vi "Build Error Message.vi"(8 "error IO":errorcluster, 9 "Enum":T1, 10 "Address":u8) -> (3 "Error Cluster":T2)   [LabVIEW 2015, in "J1939 Addon Shared.lvlib"]
uses:
  J1939 Addon Shared.lvlib
  Types/Error Cluster.ctl
  Types/Error Types.ctl
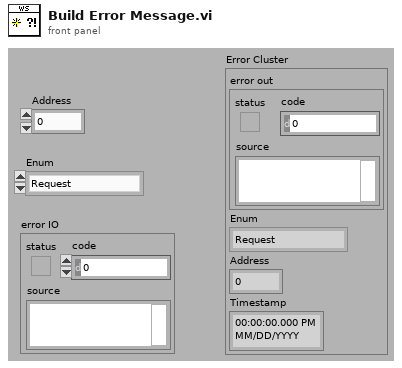
[diagram p1: front panel]
types:
  T1 = typedef "J1939 Addon Shared.lvlib/Error Types.ctl" = enum16{"Request", "RAW Generation", "Clear Active DTCs", "Clear Previous DTCs", "Addresses", "TLAs", "Get Active DTCs", "Get Previous DTCs", "TCP Connection"}
  T2 = typedef "J1939 Addon Shared.lvlib/Error Cluster.ctl" = cluster{"error out":errorcluster, "Enum":T1, "Address":u8, "Timestamp":timestamp}
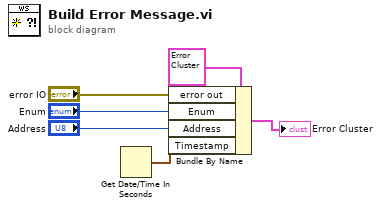
[diagram p0: block diagram]
diagram:
  n1 = Get Date/Time In Seconds() -> (seconds since 1Jan1904=w5:timestamp)
  n2 = Bundle By Name(cluster=T2 {"error out"={"status"=FALSE, "code"=0, "source"=""}, "Enum"=enum."Request", "Address"=0, "Timestamp"=timestamp(0 s since 1904-01-01)} ("Error Cluster"), "error out"="error IO", "Enum"="Enum", "Address"="Address", "Timestamp"=w5) -> (→"Error Cluster":T2)
